vi "EnumToEnum.vi"() -> ()   [LabVIEW 2024]
uses:
  <vilib>/regexp/Match Regular Expression.xnode
panel:
  in  "Enum":enum16{""}(ring)
  out "Doc":string
  in  "#Define list":string="#define SDL_WINDOW_FULLSCREEN           SDL_UINT64_C(0x0000000000000001)    /**< window is in fullscreen mode */\n#define SDL_WINDOW_OPENGL               SDL_UINT64_C(0x0000000000000002)    /**< window usable with OpenGL context */\n#define SDL_WINDOW_OCCLUDED             SDL_UINT64_C(0x0000000000000004)    /**< window is occluded */\n#define SDL_WINDOW_HIDDEN               SDL_UINT64_C(0x0000000000000008)    /**< window is neither mapped onto the desktop nor shown in the taskbar/dock/window list; SDL_ShowWindow() is required for it to become visible */\n#define SDL_WINDOW_BORDERLESS           SDL_UINT64_C(0x0000000000000010)    /**< no window decoration */\n#define SDL_WINDOW_RESIZABLE            SDL_UINT64_C(0x0000000000000020)    /**< window can be resized */\n#define SDL_WINDOW_MINIMIZED            SDL_UINT64_C(0x0000000000000040)    /**< window is minimized */\n#define SDL_WINDOW_MAXIMIZED            SDL_UINT64_C(0x0000000000000080)    /**< window is maximized */\n#define SDL_WINDOW_MOUSE_GRABBED        SDL_UINT64_C(0x0000000000000100)    /**< window has grabbed mouse input */\n#define SDL_WINDOW_INPUT_FOCUS          SDL_UINT64_C(0x0000000000000200)    /**< window has input focus */\n#define SDL_WINDOW_MOUSE_FOCUS          SDL_UINT64_C(0x0000000000000400)    /**< window has mouse focus */\n#define SDL_WINDOW_EXTERNAL             SDL_UINT64_C(0x0000000000000800)    /**< window not created by SDL */\n#define SDL_WINDOW_MODAL                SDL_UINT64_C(0x0000000000001000)    /**< window is modal */\n#define SDL_WINDOW_HIGH_PIXEL_DENSITY   SDL_UINT64_C(0x0000000000002000)    /**< window uses high pixel density back buffer if possible */\n#define SDL_WINDOW_MOUSE_CAPTURE        SDL_UINT64_C(0x0000000000004000)    /**< window has mouse captured (unrelated to MOUSE_GRABBED) */\n#define SDL_WINDOW_MOUSE_RELATIVE_MODE  SDL_UINT64_C(0x0000000000008000)    /**< window has relative mode enabled */\n#define SDL_WINDOW_ALWAYS_ON_TOP        SDL_UINT64_C(0x0000000000010000)    /**< window should always be above others */\n#define SDL_WINDOW_UTILITY              SDL_UINT64_C(0x0000000000020000)    /**< window should be treated as a utility window, not showing in the task bar and window list */\n#define SDL_WINDOW_TOOLTIP              SDL_UINT64_C(0x0000000000040000)    /**< window should be treated as a tooltip and does not get mouse or keyboard focus, requires a parent window */\n#define SDL_WINDOW_POPUP_MENU           SDL_UINT64_C(0x0000000000080000)    /**< window should be treated as a popup menu, requires a parent window */\n#define SDL_WINDOW_KEYBOARD_GRABBED     SDL_UINT64_C(0x0000000000100000)    /**< window has grabbed keyboard input */\n#define SDL_WINDOW_VULKAN               SDL_UINT64_C(0x0000000010000000)    /**< window usable for Vulkan surface */\n#define SDL_WINDOW_METAL                SDL_UINT64_C(0x0000000020000000)    /**< window usable for Metal view */\n#define SDL_WINDOW_TRANSPARENT          SDL_UINT64_C(0x0000000040000000)    /**< window with transparent buffer */\n#define SDL_WINDOW_NOT_FOCUSABLE        SDL_UINT64_C(0x0000000080000000)    /**< window should not be focusable */"
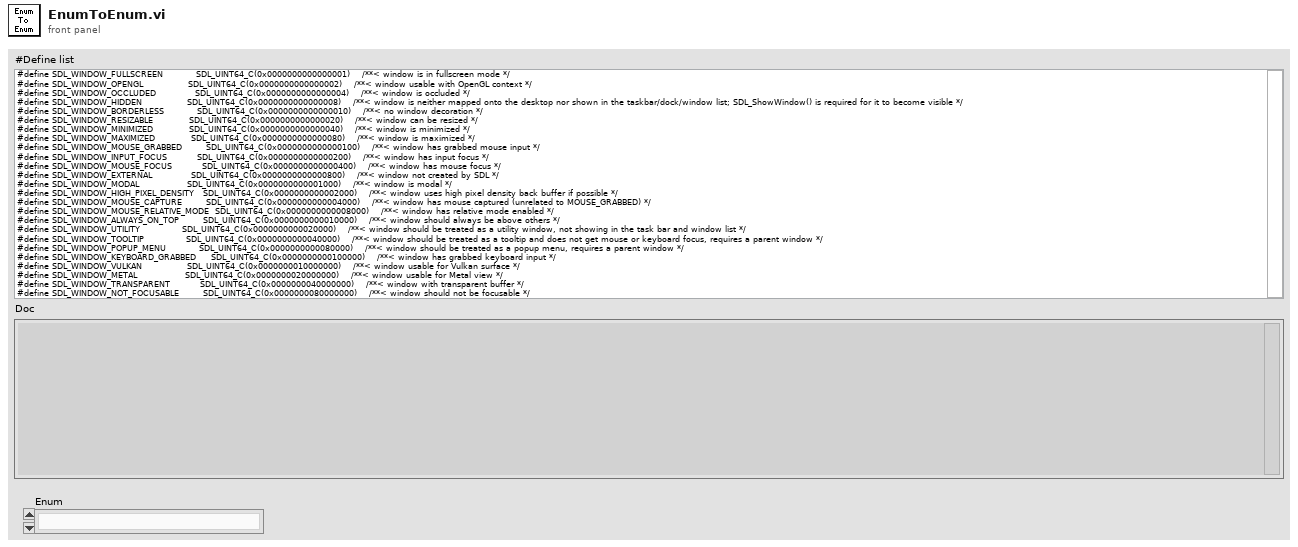
[diagram p1: front panel]
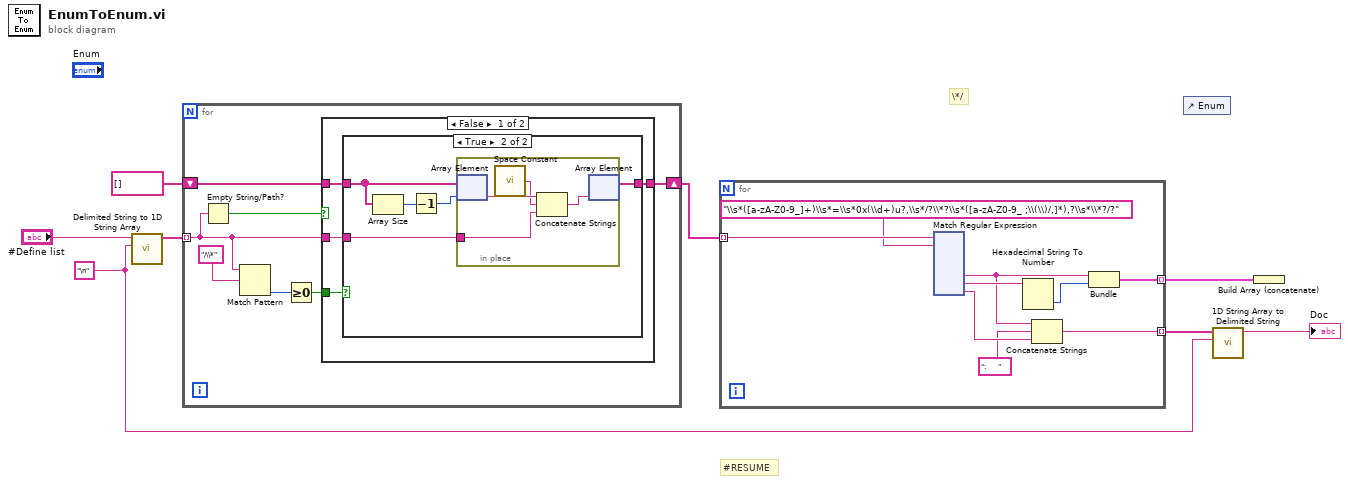
[diagram p0: block diagram]
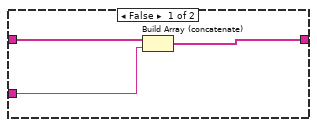
[diagram p2: hidden frame]
diagram:
  w5 = "\n" ("delimiter")
  # "#RESUME"
  # "\\*/"
  n1 = call <vilib>:"Delimited String to 1D String Array.vi"("delimiter"=w5, "delimited string"="#Define list") -> ("string array"=w3:string[])  [unwired: 9 in]
  n2 = for {
    tunnel: w3 -> [w10] mode=indexing
    shift-right: [w13] -> w1
    shift-left: string[] [] -> [w14]
    n3 = Empty String/Path?(string/path=w10) -> (empty?=w9:bool)
    n4 = Match Pattern(string=w10, regular expression="/\\*") -> (offset past match=w12:i32)  [unwired: 1 in, 3 out]
    n5 = Greater Or Equal To 0?(x=w12) -> (x >= 0?=w11:bool)
    n6 = case shown="False" w9 {
      tunnel: w14 -> [w19 w32]
      tunnel: [w18 w32] -> w13
      tunnel: w11 -> [w17 _]
      tunnel: w10 -> [w16 _]
      frame False {
        n7 = case shown="True" w17 {
          tunnel: w19 -> [w22 w27]
          tunnel: [w21 w26] -> w18
          tunnel: w16 -> [w20 w25]
          frame False {
            n8 = Build Array (concatenate)(w22, w20) -> (w21:string[])
          }
          frame True {
            n9 = Array Size(array=w27) -> (size(s)=w24:i32)
            n10 = Decrement(x=w24) -> (x-1=w23:i32)
            n11 = in-place {
              in-place-border: w25 -> [w28]
              n12 = in-place-array #1(w27, w23) -> (w31:string)
              n13 = call <vilib>:"Space Constant.vi"() -> ("String"=w29:string)
              n14 = Concatenate Strings(w31, w29, w28) -> (w30:string)
              n15 = in-place-array #1(w30) -> (w26:string[])  [unwired: 1 out]
            }
          }
        }
      }
      frame True {
      }
    }
  }
  n16 = for {
    tunnel: w1 -> [w41] mode=indexing
    tunnel: [w38] -> w7 mode=indexing
    tunnel: [w34] -> w6 mode=indexing
    n17 = xnode "Match Regular Expression"("input string"=w41, "regular expression"="\\s*([a-zA-Z0-9_]+)\\s*=\\s*0x(\\d+)u?,\\s*/?\\*?\\s*([a-zA-Z0-9_ ;\\(\\)/,]*),?\\s*\\*?/?") -> ("submatch 1"=w36:string, "submatch 2"=w39:string, "submatch 3"=w35:string)  [unwired: 4 in, 5 out]
    n18 = Hexadecimal String To Number(string=w39) -> (number=w37:u32)  [unwired: 2 in, 1 out]
    n19 = Concatenate Strings(w36, ":      " ("string"), w35) -> (w34:string)
    n20 = Bundle("submatch 1"=w36, w37) -> (w38:cluster{"submatch 1":string, u32})  [unwired: 1 in]
  }
  n21 = control-ref of="Enum"() -> ()  [unwired: 1 out]
  n22 = call <vilib>:"1D String Array to Delimited String.vi"("delimiter"=w5, "string array"=w6) -> ("delimited string"=→"Doc":string)  [unwired: 9 in]
  n23 = Build Array (concatenate)(w7) -> ()  [unwired: 1 out]
